vi "Read Instrument.vi"(8 "error in (no error)":errorcluster, 11 "Instrument Owner in":refnum<class "Instrument Owner.lvclass">) -> (0 "error out":errorcluster, 2 "Instrument out":refnum<class "Instrument Driver.lvclass">, 3 "Instrument Owner out":refnum<class "Instrument Owner.lvclass">)   [LabVIEW 2020, in "Instrument Handler.lvlib" / "Instrument Owner.lvclass"]
doc: "This VI exposes the Instrument Read to the Community Scope."
uses:
  Instrument Owner.lvclass
  PPL/HDH.Actor Framework.Core.Instrument Driver.lvlibp/Instrument Driver/Instrument Driver.lvclass
  Instrument Sequencer/Instrument Sequencer.lvclass
  Instrument Sequencer/Instrument Sequencer.lvclass/Instrument Sequencer.ctl
  PPL/HDH.Actor Framework.Core.Sequencer.lvlibp/Sequencer/Sequencer.lvclass
  C:/Current projects/WS/PPL/HDH.Actor Framework.Core.Sequencer.lvlibp/Sequencer/Sequencer.lvclass
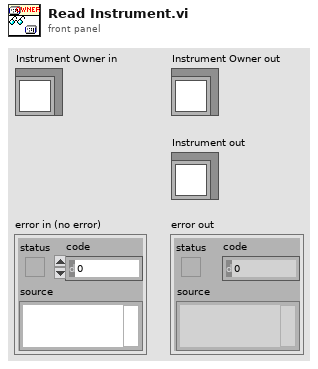
[diagram p1: front panel]
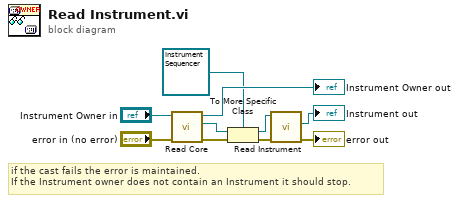
[diagram p0: block diagram]
diagram:
  # "if the cast fails the error is maintained. \nIf the Instrument owner does not contain an Instrument it should stop."
  n1 = call "Read Core.vi"("error in (no error)"="error in (no error)", "Sequencer in"="Instrument Owner in") -> ("error out"=w5:errorcluster, "Core"=w7:refnum<class "Sequencer Core.lvclass">, "Sequencer out"=→"Instrument Owner out":refnum<class "Instrument Owner.lvclass">)  [unwired: 7 in]
  n2 = To More Specific Class(target class=refnum<class "Instrument Sequencer.lvclass"> refnum ("Instrument Handler.lvlib:Instrument Sequencer.lvclass"), reference=w7, error in=w5) -> (specific class reference=w4:refnum<class "Instrument Sequencer.lvclass">, error out=w3:errorcluster)
  n3 = call "Read Instrument.vi"("error in (no error)"=w3, "Instrument Sequencer in"=w4) -> ("error out"=→"error out":errorcluster, "Instrument Driver"=→"Instrument out":refnum<class "Instrument Driver.lvclass">)  [unwired: 7 in, 1 out]
